vi "滞后.vi"(10 "检测点":dbl, 11 "XY图":cluster{dbl[], dbl[]}[](graph)) -> (2 "右滞后":dbl, 3 "左滞后":dbl)   [LabVIEW 2019]
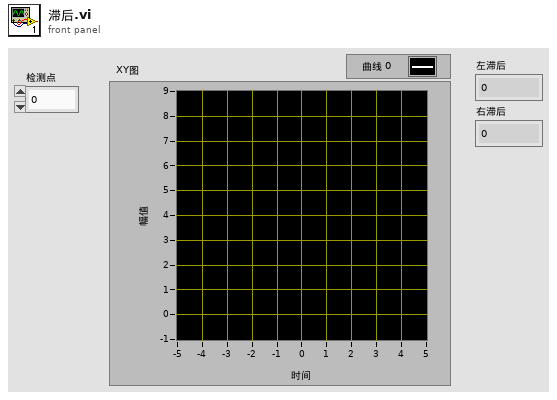
[diagram p1: front panel]
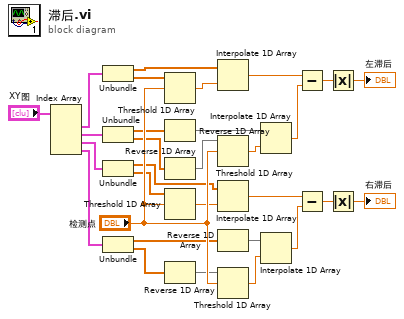
[diagram p0: block diagram]
diagram:
  n1 = Index Array(array="XY图") -> (element #1=w24:cluster{dbl[], dbl[]}, element #2=w22:cluster{dbl[], dbl[]}, element #3=w23:cluster{dbl[], dbl[]}, element #4=w21:cluster{dbl[], dbl[]})  [unwired: 4 in]
  n2 = Unbundle(w24) -> (w28:dbl[], w25:dbl[])
  n3 = Unbundle(w22) -> (w16:dbl[], w14:dbl[])
  n4 = Unbundle(w23) -> (w26:dbl[], w27:dbl[])
  n5 = Unbundle(w21) -> (w12:dbl[], w10:dbl[])
  n6 = Threshold 1D Array(2:"检测点", 3:w25) -> (0:w20:dbl)  [unwired: 1 in]
  n7 = Reverse 1D Array(array=w16) -> (reversed array=w15:dbl[])
  n8 = Reverse 1D Array(array=w14) -> (reversed array=w13:dbl[])
  n9 = Threshold 1D Array(2:"检测点", 3:w27) -> (0:w19:dbl)  [unwired: 1 in]
  n10 = Reverse 1D Array(array=w10) -> (reversed array=w9:dbl[])
  n11 = Interpolate 1D Array(1:w20, 2:w28) -> (0:w8:dbl)
  n12 = Threshold 1D Array(2:"检测点", 3:w13) -> (0:w18:dbl)  [unwired: 1 in]
  n13 = Interpolate 1D Array(1:w19, 2:w26) -> (0:w6:dbl)
  n14 = Reverse 1D Array(array=w12) -> (reversed array=w11:dbl[])
  n15 = Threshold 1D Array(2:"检测点", 3:w9) -> (0:w17:dbl)  [unwired: 1 in]
  n16 = Interpolate 1D Array(1:w18, 2:w15) -> (0:w7:dbl)
  n17 = Interpolate 1D Array(1:w17, 2:w11) -> (0:w5:dbl)
  n18 = Subtract(x=w8, y=w7) -> (x-y=w4:dbl)
  n19 = Subtract(x=w6, y=w5) -> (x-y=w2:dbl)
  n20 = Absolute Value(x=w4) -> (abs(x)=→"左滞后":dbl)
  n21 = Absolute Value(x=w2) -> (abs(x)=→"右滞后":dbl)
